vi "Toolkit Error Handling - Get API VI List.vi"(8 "error in (no error)":errorcluster) -> (0 "error out":errorcluster, 2 "API VI List":string[](array[string]))   [LabVIEW 2011]
doc: "Gets the Toolkit API VI List"
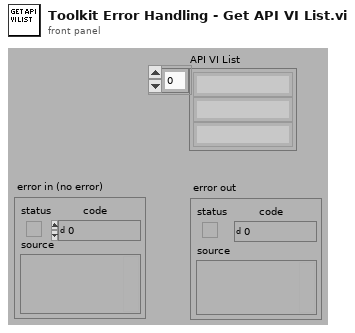
[diagram p1: front panel]
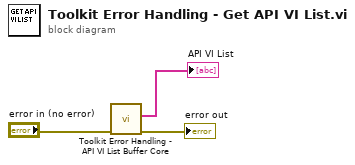
[diagram p0: block diagram]
diagram:
  n1 = call "Toolkit Error Handling - API VI List Buffer Core.vi"("error in (no error)"="error in (no error)") -> ("error out"=→"error out":errorcluster, "API VI List"=→"API VI List":string[])  [unwired: 9 in]
